vi "Obtain panel remote close event.vi"(8 "error in (no error)":errorcluster, 11 "Fiber Auto Collimation panel":refnum<class "Fiber Auto Collimation panel.lvclass">) -> (0 "error out":errorcluster, 3 "Panel remote close":refnum<user-event>)   [LabVIEW 2018, in "Fiber Auto Collimation References.lvclass"]
doc: "This VI gets the reference to an event that tells any panel to close, if it's registered for this event.\n\nAll panels except the Apex and Main panel should register for this event in order to close themselves when it is received unless there is a specific reason NOT to do so.\n\nThis event is created specifically for each class AND each clone (if cloneable). If this event is generated with a class passed in that is not running, or is running but doesn't match the clone name exactly, nothing will happen. The class data is passed along so that if a panel wants to have some meta-information passed on inside the event, it can, but by default just the generation of the event is all that is needed to trigger the close.\n\nBecause this event is created once per panel and once per clone, it should be destroyed right before the panel finally closes to avoid memory leaks."
uses:
  Fiber Auto Collimation References.lvclass
  Panels/Fiber Auto Collimation panel.lvclass
  C:/Program Files (x86)/National Instruments/LabVIEW 2018/user.lib/nLight Tidbits/Cross-library references/Cross-library key/Cross-library key.lvclass
  b47026bc-8271-46ff-bcce-21c2580a6587.vi
  f406f5ab-9891-41e2-b0a1-c13e850666b3.vi
  b47026bc-8271-46ff-bcce-21c2580a6587.vi/80a55534-07b4-46f3-95dc-9cfd723c105d.vi
  <userlib>/nLight Tidbits/Cross-library references/Cross-library key/Obtain cross library semaphore and acquire.vi
  b47026bc-8271-46ff-bcce-21c2580a6587.vi/4da48868-7ba5-4708-8795-12157d94ca14.vi
  f406f5ab-9891-41e2-b0a1-c13e850666b3.vi/53d4c5d6-f8c1-450b-89f8-0892ad8fc76d.vi
  f406f5ab-9891-41e2-b0a1-c13e850666b3.vi/861b9ba3-e80f-41d3-82b8-501c193dd8d2.vi
  <userlib>/nLight Error Handling/Trash error.vi
  <vilib>/Utility/error.llb/Clear Errors.vi
  <vilib>/Utility/semaphor.llb/Obtain Semaphore Reference.vi
  <vilib>/Utility/semaphor.llb/Acquire Semaphore.vi
  <userlib>/nLight Error Handling/Log any errors.vi
  <userlib>/nLight Tidbits/Cross-library references/Cross-library key/Obtain class key.vi
  <vilib>/Utility/semaphor.llb/Release Semaphore.vi
  <vilib>/Utility/semaphor.llb/Release Semaphore Reference.vi
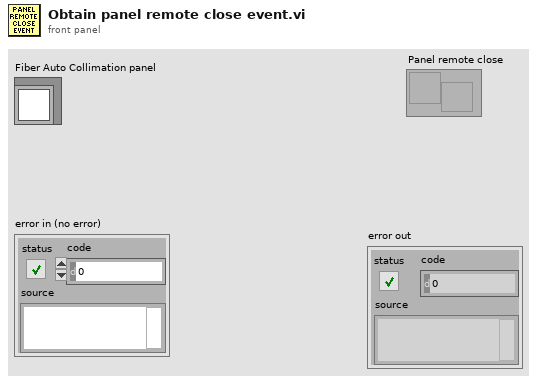
[diagram p1: front panel]
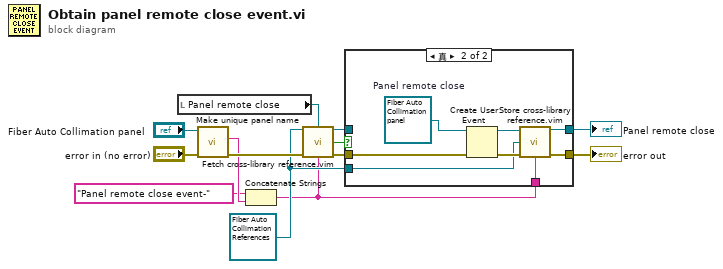
[diagram p0: block diagram]
diagram:
  w8 = refnum<class "Fiber Auto Collimation References.lvclass"> refnum ("nLight Station Template References.lvclass")
  n1 = local read "Panel remote close"() -> (w9:refnum<user-event>)
  n2 = call "Make unique panel name.vi"("error in (no error)"="error in (no error)", "Fiber Auto Collimation panel in"="Fiber Auto Collimation panel") -> ("error out"=w10:errorcluster, "Unique panel name"=w5:string)  [unwired: 7 in, 1 out]
  n3 = Concatenate Strings("Panel remote close event-" ("string"), w5) -> (w4:string)
  n4 = call "Fetch cross-library reference.vim"("Cross-library key"=w8, "Reference type to fetch"=w9, "error in (no error)"=w10, "Specific ref type name [String/Enum]"=w4) -> ("Stored value (if present)"=w1:refnum<user-event>, "Nothing to fetch OR bad reference"=w7:bool, "error out"=w6:errorcluster)  [unwired: 9 in]
  n5 = case shown="真" w7 {
    tunnel: w6 -> [w15 w23]
    tunnel: [w15 w19] -> w13
    tunnel: [w14 w20] -> w2
    tunnel: w8 -> [_ w18]
    tunnel: w4 -> [_ w17]
    tunnel: w1 -> [w14 _]
    frame False {
    }
    frame True {
      w16 = refnum<class "Fiber Auto Collimation panel.lvclass"> refnum  # Panel remote close
      n6 = Create User Event(user event datatype=w16, error in=w23) -> (user event=w21:refnum<user-event>, error out=w22:errorcluster)
      n7 = call "Store cross-library reference.vim"("Reference to store"=w21, "Cross-library key"=w18, "error in (no error)"=w22, "Specific ref type name [String/Enum]"=w17) -> ("Copy of stored reference"=w20:refnum<user-event>, "error out"=w19:errorcluster)  [unwired: 8 in, 2 out]
    }
  }
  "error out" <- w13
  "Panel remote close" <- w2
